vi "Find Turn Error.vi"(0 "Target Angle":dbl, 3 "Current Angle":dbl) -> (7 "Error":dbl)   [LabVIEW 2016]
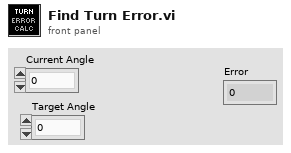
[diagram p1: front panel]
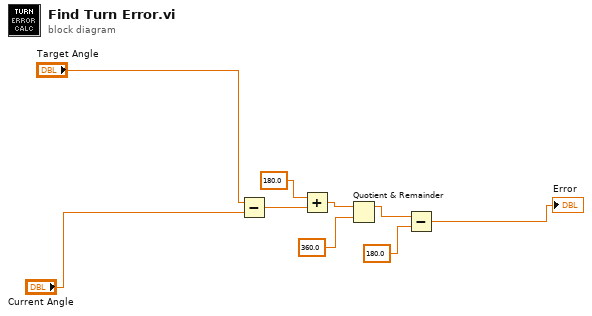
[diagram p0: block diagram]
diagram:
  n1 = Subtract(x="Target Angle", y="Current Angle") -> (x-y=w9:dbl)
  n2 = Add(x=180.0, y=w9) -> (x+y=w7:dbl)
  n3 = Quotient & Remainder(x=w7, y=360.0) -> (x-y*floor(x/y)=w5:dbl)  [unwired: 1 out]
  n4 = Subtract(x=w5, y=180.0) -> (x-y=→"Error":dbl)
